vi "Broadcast Commands.vi"() -> ()   [LabVIEW 2020]
doc: "This example demostrates how to use UDP with STM to broadcast messages to multiple systems at once.\n\nThe \"Listen and Acknowledge Commands\" VI must be started first.\n\nCopyright 2015, 2016, 2017 National Instruments Corporation\n\nLicensed under the Apache License, Version 2.0 (the \"License\"); you may not use this file except in compliance with the License.\n\n You may obtain a copy of the License at\n\n http://www.apache.org/licenses/LICENSE-2.0\n\nUnless required by applicable law or agreed to in writing, software distributed under the License is distributed on an \"AS IS\" BASIS, WITHOUT WARRANTIES OR CONDITIONS OF ANY KIND, either express or implied.\n\nSee the License for the specific language governing permissions and limitations under the License."
uses:
  <vilib>/NI/STM/SubVIs/MetaDataElement.ctl
  <vilib>/NI/STM/UDP/UDP Read Options.ctl
  <vilib>/NI/STM/UDP/Write Meta Data (UDP Ref).vi
  <vilib>/NI/STM/UDP/Get Connection Reference (UDP).vi
  <vilib>/NI/STM/UDP/Write Meta Data (UDP Clst).vi
  <vilib>/NI/STM/UDP/Write Message (UDP).vi
  <vilib>/NI/STM/UDP/Read Message (UDP).vi
  <vilib>/NI/STM/NI STM.lvlib
panel:
  in  "timeout for ACK":i32=1000
  out "error out":errorcluster
  out "IP addresses who acknowledge command":string[](array[string])
  in  "Stop This App":bool
  in  "Stop":bool
  in  "Start":bool
  in  "Configure":bool
  in  "local port":u16=61556
  in  "remote port":u16=61557
  # "Commands to send"
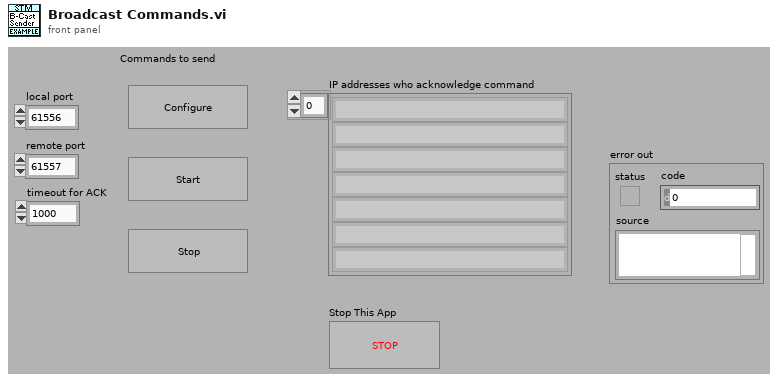
[diagram p1: front panel]
types:
  T1 = typedef "NI STM.lvlib/MetaDataElement.ctl" = string
  T2 = typedef "NI STM.lvlib/UDP Connection Info.ctl" = cluster{"connection ID":refnum<k16>, "meta data":T1[]}
  T3 = typedef "NI STM.lvlib/UDP Read Options.ctl" = cluster{"ignore timeout error":bool, "timeout ms (1000)":i32, "max size (548)":i32}
  T4 = typedef "NI STM.lvlib/UDP Data Info.ctl" = cluster{"address":u32, "port":u16, "bytes read":i32}
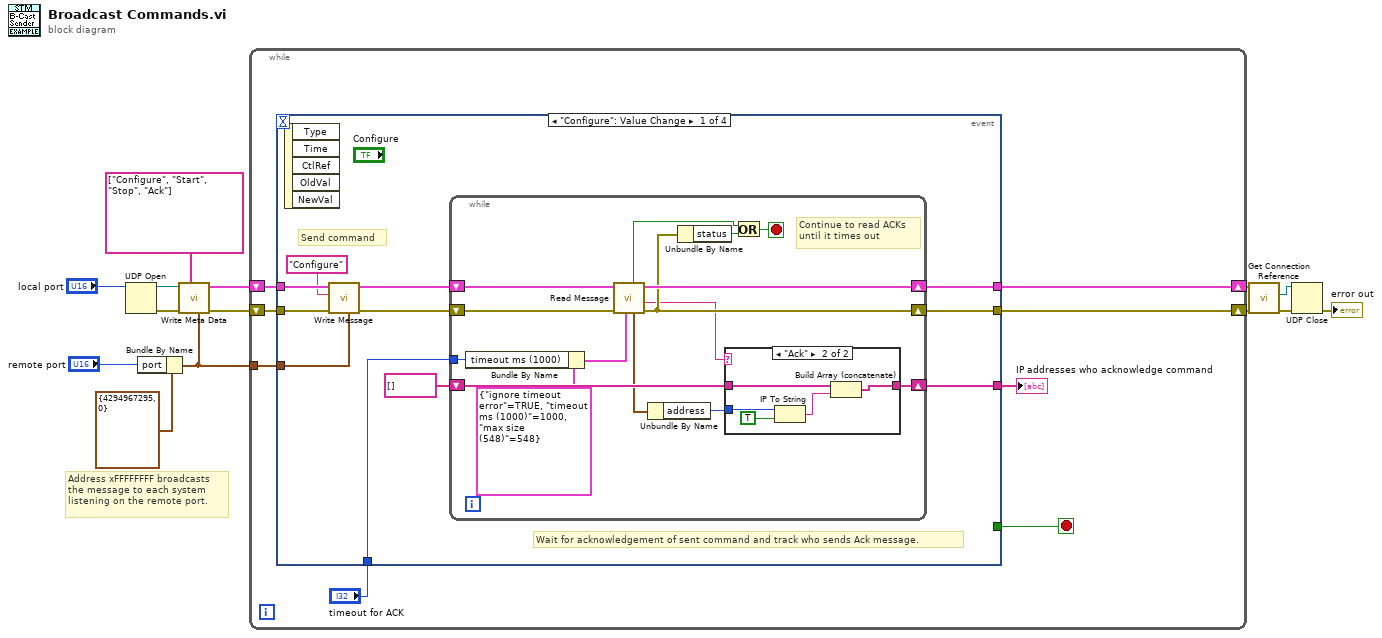
[diagram p0: block diagram]
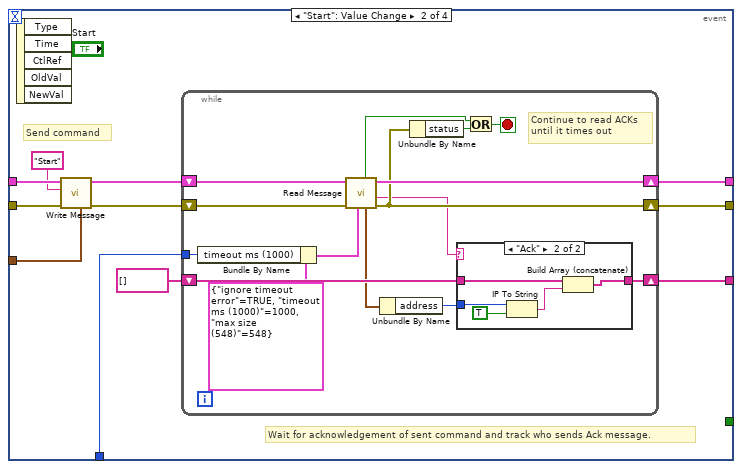
[diagram p3: hidden frame]
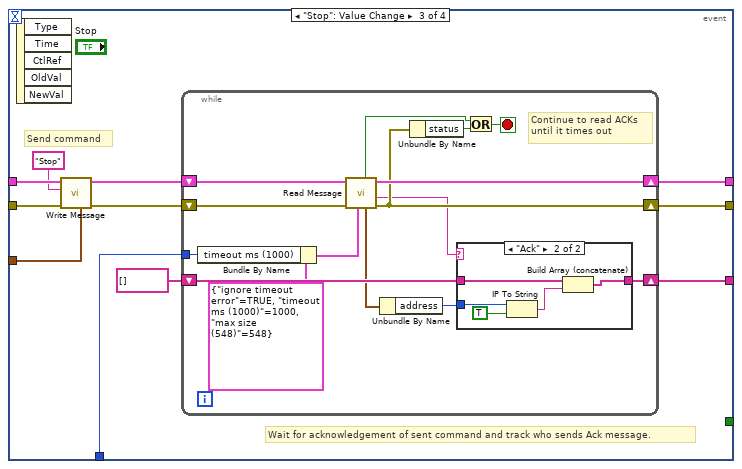
[diagram p5: hidden frame]
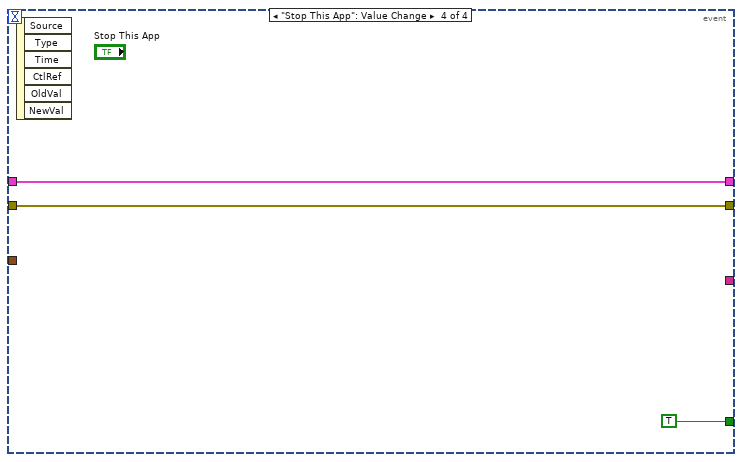
[diagram p7: hidden frame]
diagram:
  # "Address xFFFFFFFF broadcasts\nthe message to each system\nlistening on the remote port."
  n1 = UDP Open(11:"local port") -> (port=w9:refnum<k16>, 0:w12:errorcluster)  [unwired: 1 in, 4 out]
  n2 = Bundle By Name(cluster=cluster{"address":u32, "port":u16} {"address"=4294967295, "port"=0} ("Address"), "port"="remote port") -> (w6:cluster{"address":u32, "port":u16})
  n3 = call-poly <vilib>:"Write Meta Data.vi"("address"=w6, "meta data"=T1[] ["Configure", "Start", "Stop", "Ack"] ("Meta data"), "error in"=w12, "connection ID"=w9) -> ("error out"=w11:errorcluster, "connection info out"=w14:T2)  [unwired: 3 in, 3 out]
  n4 = while {
    tunnel: w6 -> [w20]
    shift-right: [w18] -> w4
    shift-left: w11 -> [w21]
    shift-right: [w17] -> w3
    shift-left: w14 -> [w22]
    stop <- w19 stop-if-true
    n5 = event shown="[0] \"Configure\": Value Change" {
      selector: _ -> [_ _ _ _]
      dyn-events: _ -> [_ _ _ _]
      timeout: _ -> [_ _ _ _]
      tunnel: w22 -> [w33 w65 w97 w120]
      tunnel: w21 -> [w32 w64 w96 w119]
      tunnel: w20 -> [w31 w63 w95 _]
      tunnel: [_ _ _ TRUE] -> w19
      tunnel: [w27 w57 w92 w119] -> w18
      tunnel: [w26 w58 w91 w120] -> w17
      tunnel: [w24 w56 w87 _] -> w16
      tunnel: "timeout for ACK" -> [w23 w55 w88 _]
      event "Configure": Value Change {
        # "Wait for acknowledgement of sent command and track who sends Ack message."
        # "Send command"
        n6 = event-data() -> ()  [unwired: 6 out]
        n7 = call-poly <vilib>:"Write Message.vi"("address"=w31, "error in"=w32, "name"="Configure" ("Name"), "connection info in"=w33) -> ("error out"=w29:errorcluster, "connection info out"=w30:T2)  [unwired: 2 in, 4 out]
        n8 = while {
          shift-right: [w43] -> w24
          shift-left: string[] [] -> [w44]
          tunnel: w23 -> [w36]
          shift-right: [w47] -> w26
          shift-left: w30 -> [w39]
          shift-right: [w45] -> w27
          shift-left: w29 -> [w48]
          stop <- w46 stop-if-true
          # "Continue to read ACKs\nuntil it times out"
          n9 = Bundle By Name(cluster=T3 {"ignore timeout error"=TRUE, "timeout ms (1000)"=1000, "max size (548)"=548} ("Options"), "timeout ms (1000)"=w36) -> (w37:T3)
          n10 = call-poly <vilib>:"Read Message.vi"("options"=w37, "error in"=w48, "connection info in"=w39) -> ("error out"=w45:errorcluster, "name"=w40:T1, "connection info out"=w47:T2, "data info"=w42:T4, "timed out?"=w34:bool)  [unwired: 1 in, 3 out]
          n11 = Unbundle By Name(w42) -> ("address"=w41:u32)
          n12 = Unbundle By Name(w45) -> ("status"=w35:bool)
          n13 = case shown="\"Ack\"" w40 {
            tunnel: w44 -> [w49 w53]
            tunnel: w41 -> [_ w51]
            tunnel: [w49 w50] -> w43
            frame "False", Default {
            }
            frame "Ack" {
              n14 = IP To String(1:TRUE ("dot notation? (F)"), 2:w51) -> (0:w52:string)
              n15 = Build Array (concatenate)(w53, w52) -> (w50:string[])
            }
          }
          n16 = Or(x=w34, y=w35) -> (x .or. y?=w46:bool)
        }
      }
      event "Start": Value Change {
        # "Wait for acknowledgement of sent command and track who sends Ack message."
        # "Send command"
        n17 = event-data() -> ()  [unwired: 6 out]
        n18 = call-poly <vilib>:"Write Message.vi"("address"=w63, "error in"=w64, "name"="Start" ("Name"), "connection info in"=w65) -> ("error out"=w59:errorcluster, "connection info out"=w60:T2)  [unwired: 2 in, 4 out]
        n19 = while {
          shift-right: [w75] -> w56
          shift-left: string[] [] -> [w76]
          tunnel: w55 -> [w68]
          shift-right: [w79] -> w58
          shift-left: w60 -> [w71]
          shift-right: [w77] -> w57
          shift-left: w59 -> [w80]
          stop <- w78 stop-if-true
          # "Continue to read ACKs\nuntil it times out"
          n20 = Bundle By Name(cluster=T3 {"ignore timeout error"=TRUE, "timeout ms (1000)"=1000, "max size (548)"=548} ("Options"), "timeout ms (1000)"=w68) -> (w69:T3)
          n21 = call-poly <vilib>:"Read Message.vi"("options"=w69, "error in"=w80, "connection info in"=w71) -> ("error out"=w77:errorcluster, "name"=w72:T1, "connection info out"=w79:T2, "data info"=w74:T4, "timed out?"=w66:bool)  [unwired: 1 in, 3 out]
          n22 = Unbundle By Name(w74) -> ("address"=w73:u32)
          n23 = Unbundle By Name(w77) -> ("status"=w67:bool)
          n24 = case shown="\"Ack\"" w72 {
            tunnel: w76 -> [w81 w85]
            tunnel: w73 -> [_ w83]
            tunnel: [w81 w82] -> w75
            frame "False", Default {
            }
            frame "Ack" {
              n25 = IP To String(1:TRUE ("dot notation? (F)"), 2:w83) -> (0:w84:string)
              n26 = Build Array (concatenate)(w85, w84) -> (w82:string[])
            }
          }
          n27 = Or(x=w66, y=w67) -> (x .or. y?=w78:bool)
        }
      }
      event "Stop": Value Change {
        # "Wait for acknowledgement of sent command and track who sends Ack message."
        # "Send command"
        n28 = event-data() -> ()  [unwired: 6 out]
        n29 = call-poly <vilib>:"Write Message.vi"("address"=w95, "error in"=w96, "name"="Stop" ("Name"), "connection info in"=w97) -> ("error out"=w89:errorcluster, "connection info out"=w90:T2)  [unwired: 2 in, 4 out]
        n30 = while {
          shift-right: [w107] -> w87
          shift-left: string[] [] -> [w108]
          tunnel: w88 -> [w100]
          shift-right: [w111] -> w91
          shift-left: w90 -> [w103]
          shift-right: [w109] -> w92
          shift-left: w89 -> [w112]
          stop <- w110 stop-if-true
          # "Continue to read ACKs\nuntil it times out"
          n31 = Bundle By Name(cluster=T3 {"ignore timeout error"=TRUE, "timeout ms (1000)"=1000, "max size (548)"=548} ("Options"), "timeout ms (1000)"=w100) -> (w101:T3)
          n32 = call-poly <vilib>:"Read Message.vi"("options"=w101, "error in"=w112, "connection info in"=w103) -> ("error out"=w109:errorcluster, "name"=w104:T1, "connection info out"=w111:T2, "data info"=w106:T4, "timed out?"=w98:bool)  [unwired: 1 in, 3 out]
          n33 = Unbundle By Name(w106) -> ("address"=w105:u32)
          n34 = Unbundle By Name(w109) -> ("status"=w99:bool)
          n35 = case shown="\"Ack\"" w104 {
            tunnel: w108 -> [w113 w117]
            tunnel: w105 -> [_ w115]
            tunnel: [w113 w114] -> w107
            frame "False", Default {
            }
            frame "Ack" {
              n36 = IP To String(1:TRUE ("dot notation? (F)"), 2:w115) -> (0:w116:string)
              n37 = Build Array (concatenate)(w117, w116) -> (w114:string[])
            }
          }
          n38 = Or(x=w98, y=w99) -> (x .or. y?=w110:bool)
        }
      }
      event "Stop This App": Value Change {
        n39 = event-data() -> ()  [unwired: 7 out]
      }
    }
    "IP addresses who acknowledge command" <- w16
  }
  n40 = call-poly <vilib>:"Get Connection Reference.vi"("error in"=w4, "connection info in"=w3) -> ("error out"=w5:errorcluster, "connection ID"=w2:refnum<k16>)  [unwired: 8 out]
  n41 = UDP Close(connection ID=w2, 8:w5) -> (error out=→"error out":errorcluster)  [unwired: 1 out]
